vi "FG Watchdog Dishes.vi"(1 "FG Action (Read)":T1, 2 "Watchdog dishes in":bool[](array[boolean])) -> (0 "Watchdog dishes out":bool[](array[boolean]))   [LabVIEW 2009]
uses:
  Actions for FG's.ctl
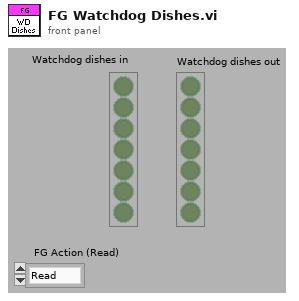
[diagram p1: front panel]
types:
  T1 = typedef "Actions for FG's.ctl" = enum16{"Read", "Write"}
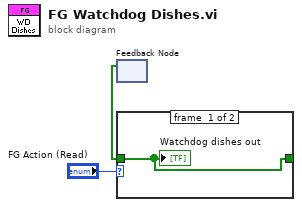
[diagram p0: block diagram]
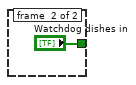
[diagram p2: hidden frame]
diagram:
  n1 = feedback #1() -> (w1:bool[])  [unwired: 1 in]
  n2 = case shown="\"Read\", Default" "FG Action (Read)" {
    tunnel: [w4 "Watchdog dishes in"] -> w2
    tunnel: w1 -> [w4 _]
    frame #0 {
      "Watchdog dishes out" <- w4
    }
    frame #1 {
    }
  }
